vi "Debug to Dashboard.vi"(10 "NT String Label":string, 11 "input":dbl) -> ()   [LabVIEW 2018]
uses:
  <vilib>/Rock Robotics/Network Tables/NT Write String.vi
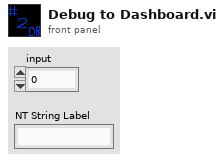
[diagram p1: front panel]
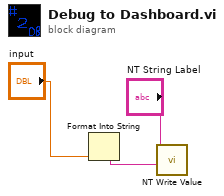
[diagram p0: block diagram]
diagram:
  n1 = Format Into String("input") -> (resulting string=w2:string)  [unwired: 3 in, 1 out]
  n2 = call-poly <vilib>:"NT Write Value.vi"("String"=w2, "Name"="NT String Label") -> ()  [unwired: 9 in, 1 out]
